vi "Swerve Drive.vi"() -> ()   [LabVIEW 2020]
panel:
  in  "W4 Encoder":dbl
  in  "W3 Encoder":dbl
  in  "W2 Encoder":dbl
  in  "W1 Encoder":dbl
  out "WS 3":dbl
  out "WS 4":dbl
  out "WS 2":dbl
  out "WS 1":dbl
  out "WA 3":dbl
  out "WA 4":dbl
  out "WA 2":dbl
  out "WA 1":dbl
  in  "RCW":dbl(slide) scale=-1.0..1.0
  in  "STR":dbl(slide) scale=-1.0..1.0
  in  "FWD":dbl(slide) scale=-1.0..1.0
  in  "Gyro":dbl
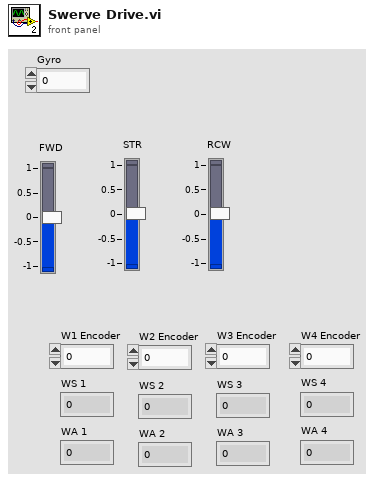
[diagram p1: front panel]
types:
  T1 = typedef "WPI_JoystickDevRef.ctl" = cluster{"Device":T2}
  T2 = typedef "WPI_JoystickDeviceEnum.ctl" = enum16{"USB 0", "USB 1", "USB 2", "USB 3", "USB 4", "USB 5"}
  T3 = typedef "WPI_MotorControlDeviceRef.ctl" = cluster{"DeviceStatus":errorcluster, "Type":T4, "PWM":cluster{"PWM Channel":T5, "DeadBand":T6}, "CAN":cluster{"Device Number":u8, "SetOutput VI Ref":variant, "GetOutput VI Ref":variant, "Enable VI Ref":variant, "Disable VI Ref":variant, "Data":variant}, "Invert":bool, "DIO PWM":cluster{"PWM \"Enable\" Channel":T5, "DIOChannel":T7, "PWM Rate":dbl}}
  T4 = typedef "WPI_MotorControlType.ctl" = enum16{"PWM", "CAN", "DIO PWM"}
  T5 = typedef "FPGA_DIOPWMChannel.ctl" = enum8{"PWM 0", "PWM 1", "PWM 2", "PWM 3", "PWM 4", "PWM 5", "PWM 6", "PWM 7", "PWM 8", "PWM 9", "PWM MXP 0", "PWM MXP 1", "PWM MXP 2", "PWM MXP 3", "PWM MXP 4", "PWM MXP 5", "PWM MXP 6", "PWM MXP 7", "PWM MXP 8", "PWM MXP 9", "Invalid"}
  T6 = typedef "WPI_PWMDeadband.ctl" = cluster{"Name":string, "maxPositivePwm":i32, "minPositivePwm":i32, "centerPwm":i32, "maxNegativePwm":i32, "minNegativePwm":i32, "angularRange":u16}
  T7 = typedef "FPGA_DIOChannel.ctl" = enum8{"DIO 0", "DIO 1", "DIO 2", "DIO 3", "DIO 4", "DIO 5", "DIO 6", "DIO 7", "DIO 8", "DIO 9", "DIO MXP 0", "DIO MXP 1", "DIO MXP 2", "DIO MXP 3", "DIO MXP 4", "DIO MXP 5", "DIO MXP 6", "DIO MXP 7", "DIO MXP 8", "DIO MXP 9", "DIO MXP 10", "DIO MXP 11", "DIO MXP 12", "DIO MXP 13", "DIO MXP 14", "DIO MXP 15", "SPI Port CS1", "SPI Port CS2", "SPI Port CS3", "SPI Port MISO", "SPI Port MOSI", "Invalid"}
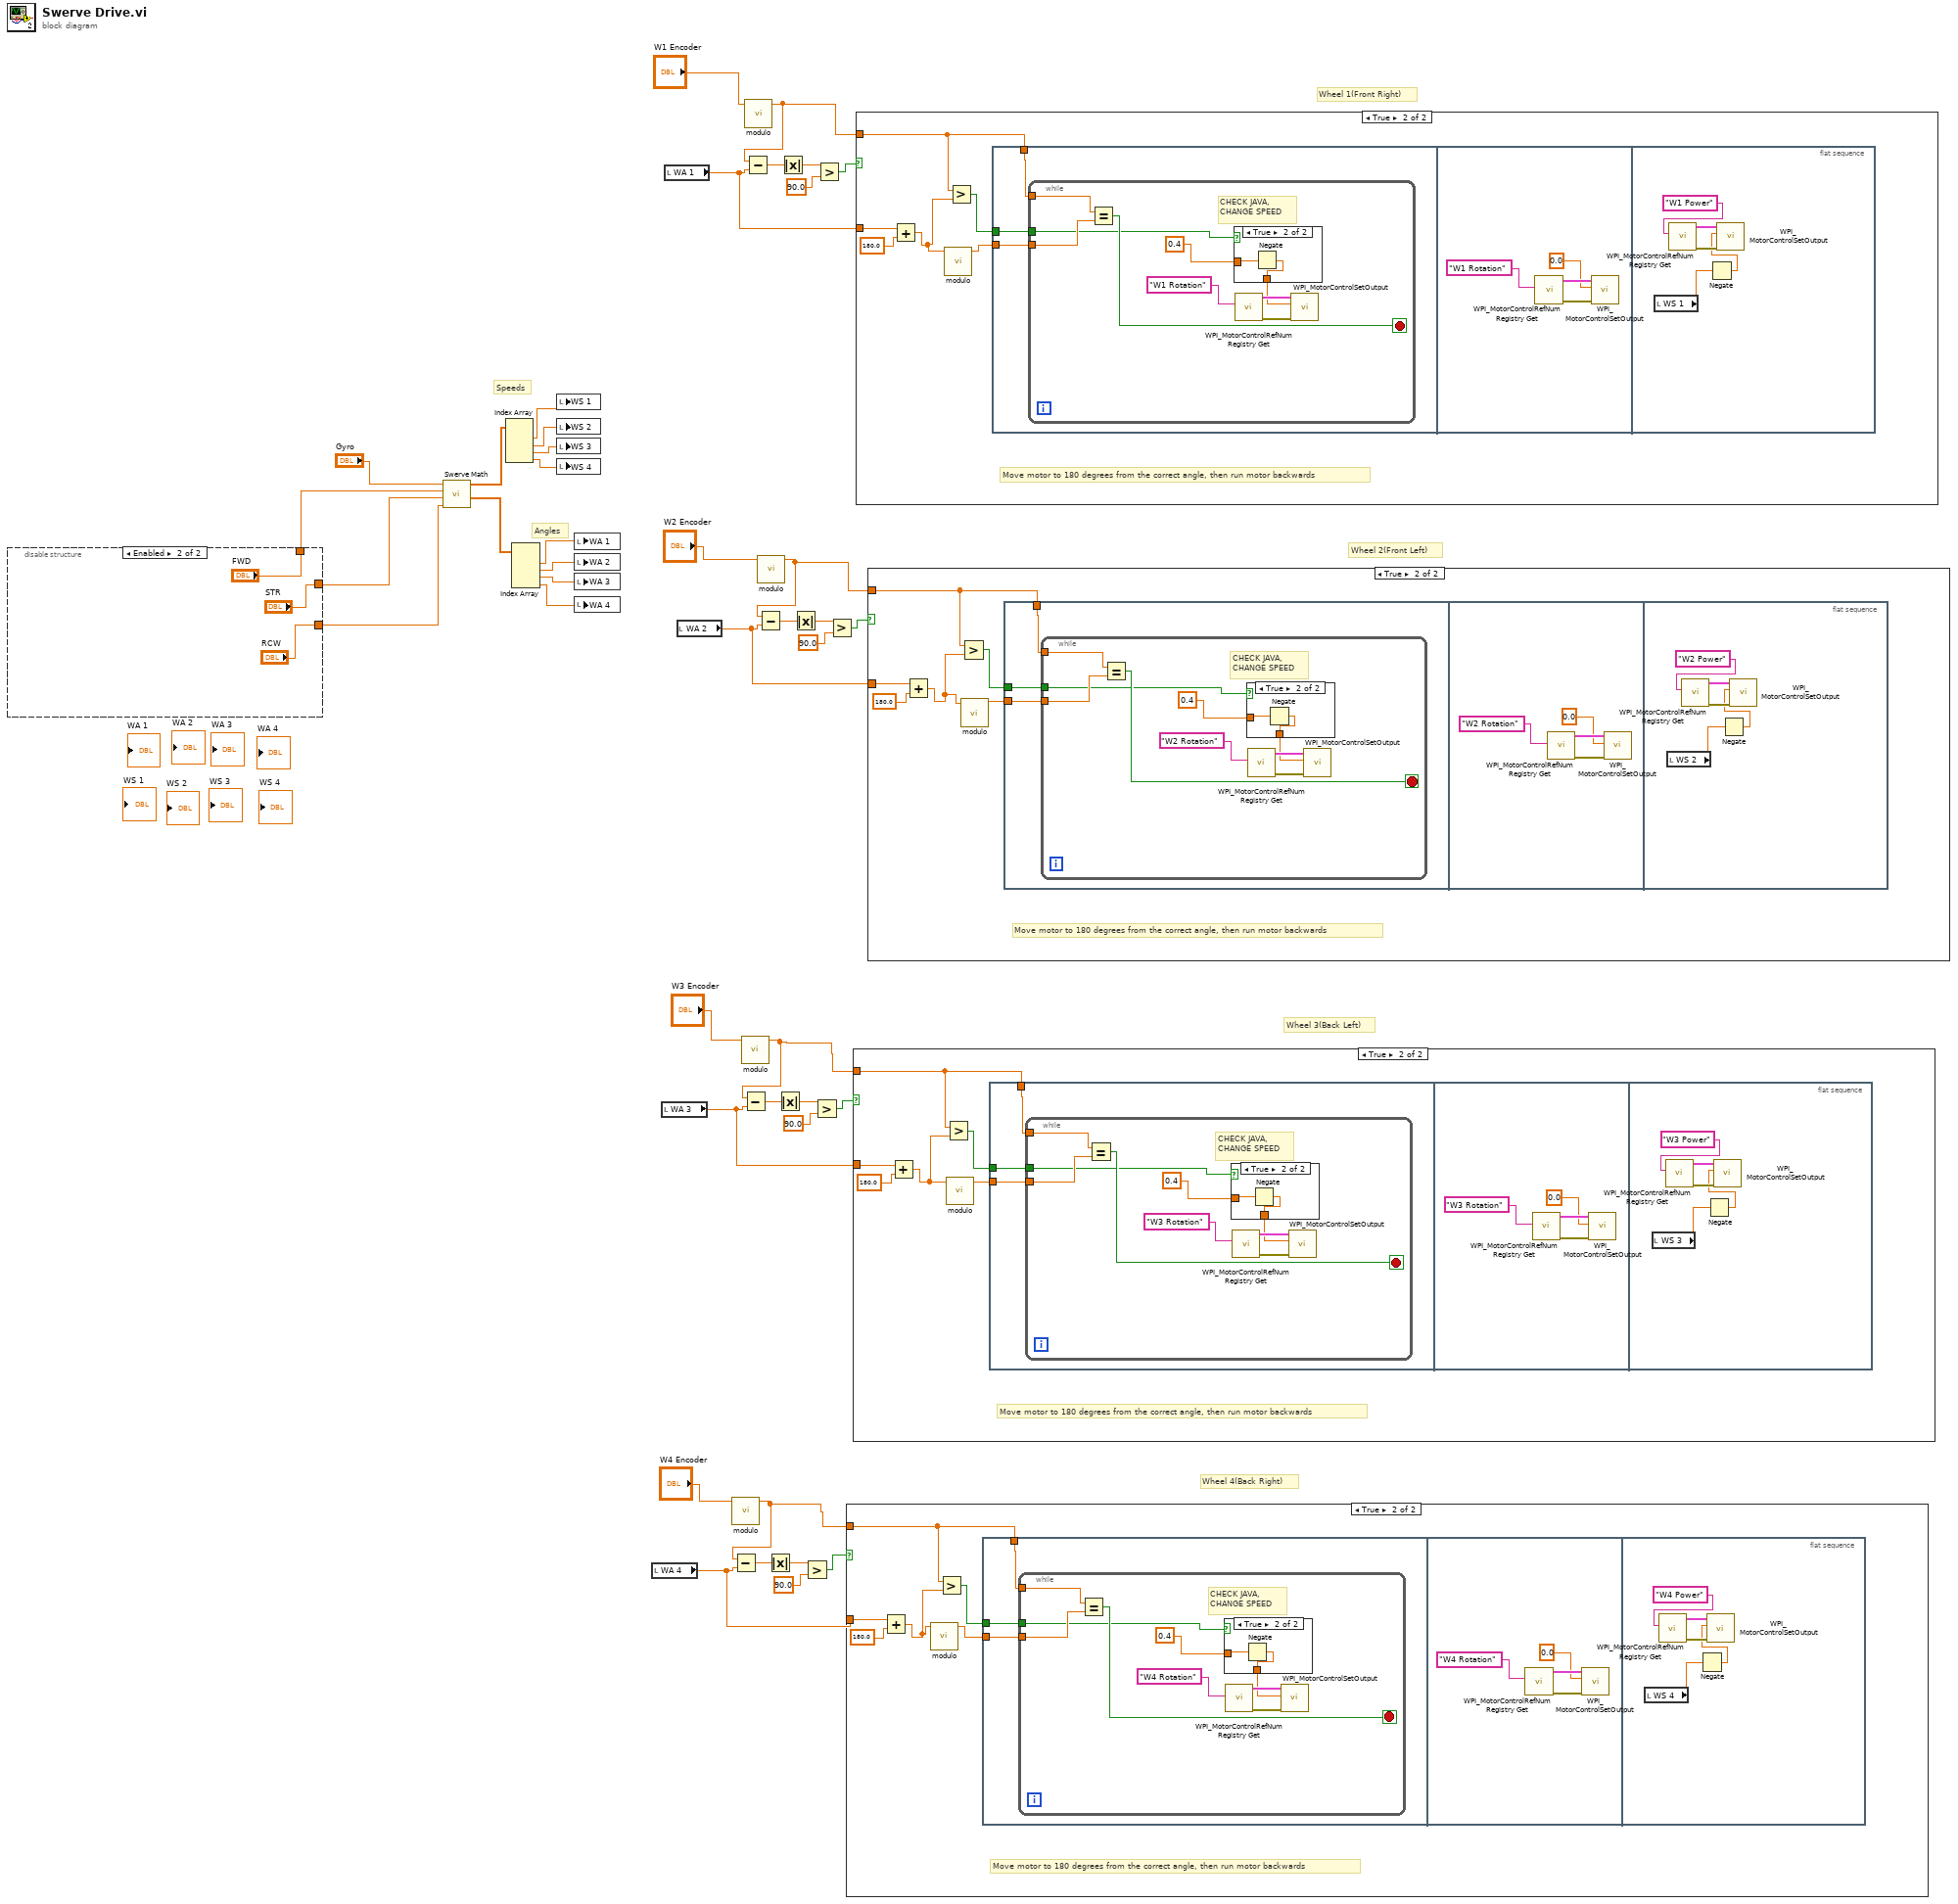
[diagram p0: block diagram]
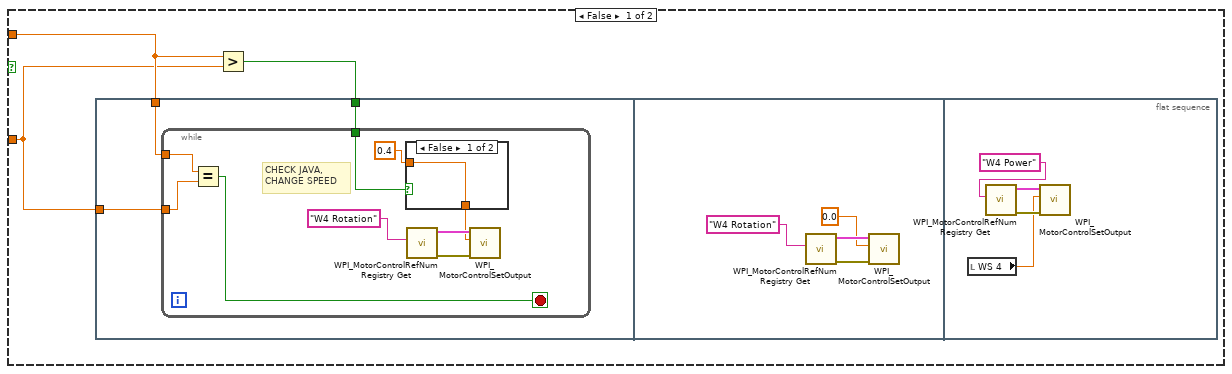
[diagram p2: hidden frame]
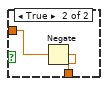
[diagram p3: hidden frame]
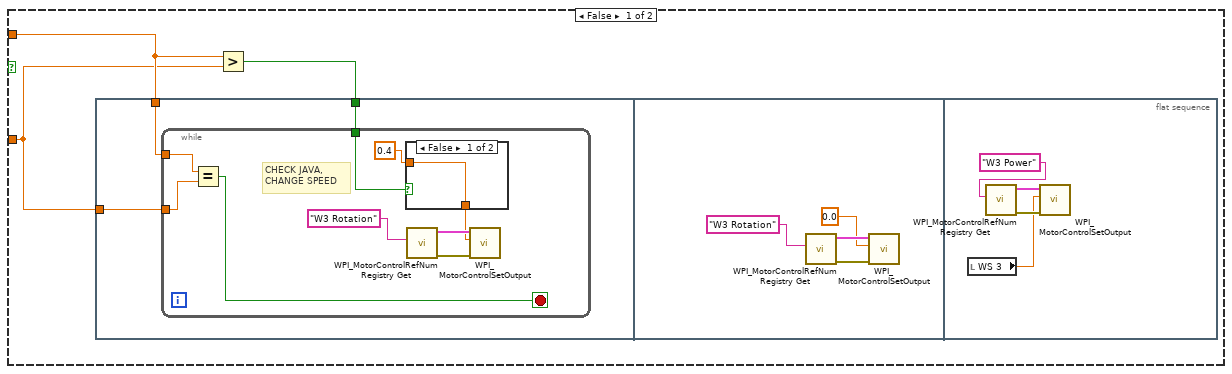
[diagram p5: hidden frame]
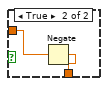
[diagram p6: hidden frame]
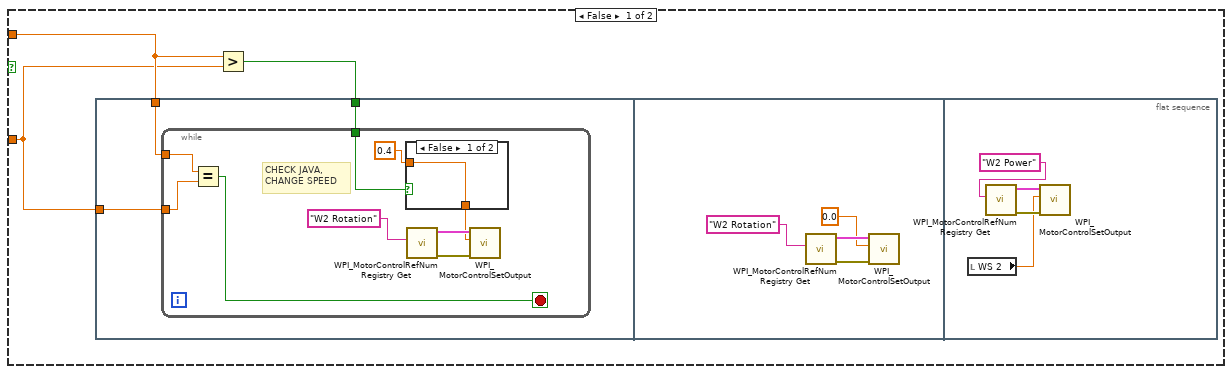
[diagram p8: hidden frame]
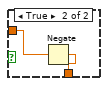
[diagram p9: hidden frame]
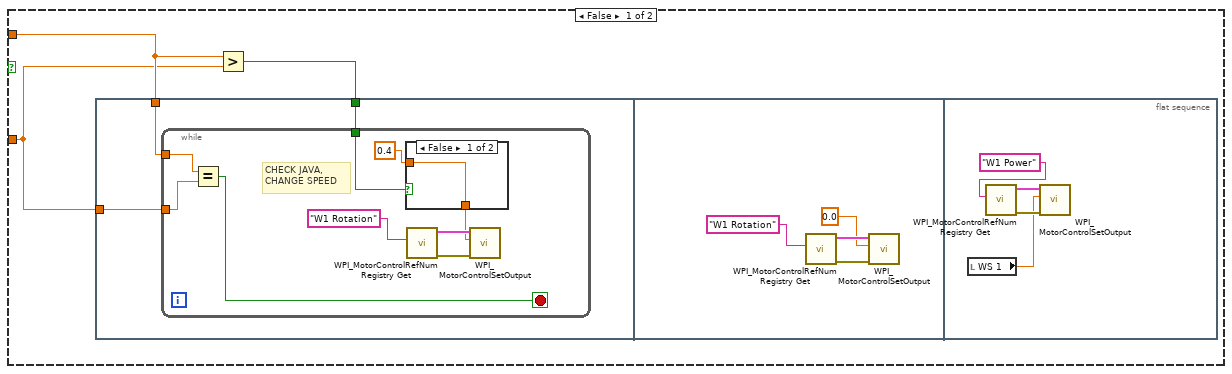
[diagram p11: hidden frame]
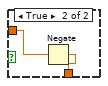
[diagram p12: hidden frame]
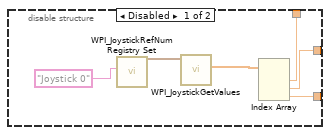
[diagram p14: hidden frame]
diagram:
  # "Wheel 4(Back Right)"
  # "Wheel 3(Back Left)"
  # "Wheel 2(Front Left)"
  # "Wheel 1(Front Right)"
  # "Angles"
  # "Speeds"
  n1 = disable-structure shown="Enabled" {
    disable-tunnel: [w45 "STR"] -> w41
    disable-tunnel: [w44 "RCW"] -> w40
    disable-tunnel: [w43 "FWD"] -> w39
    frame Disabled {
      n2 = call <vilib>:"WPI_JoystickRefNum Registry Set.vi"("refnum name"="Joystick 0") -> ("JoystickDevRef"=w47:T1)  [unwired: 9 in, 1 out]
      n3 = call <vilib>:"WPI_JoystickGetValues.vi"("JoystickDevRef"=w47) -> ("Axes"=w46:dbl[])  [unwired: 6 in, 4 out]
      n4 = Index Array(array=w46) -> (element #1=w43:dbl, element #2=w45:dbl, element #3=w44:dbl)  [unwired: 3 in]
    }
    frame Enabled {
    }
  }
  n5 = call "Swerve Math.vi"("Gyro"="Gyro", "FWD"=w39, "STR"=w41, "RCW"=w40) -> ("Wheel Speeds"=w38:dbl[], "Wheel Angles"=w37:dbl[])  [unwired: 5 in]
  n6 = Index Array(array=w38) -> (element #1=w36:dbl, element #2=w34:dbl, element #3=w35:dbl, element #4=w33:dbl)  [unwired: 4 in]
  n7 = Index Array(array=w37) -> (element #1=w29:dbl, element #2=w30:dbl, element #3=w32:dbl, element #4=w31:dbl)  [unwired: 4 in]
  n8 = local write "WS 1"(w36) -> ()
  n9 = local write "WS 2"(w34) -> ()
  n10 = local write "WS 3"(w35) -> ()
  n11 = local write "WS 4"(w33) -> ()
  n12 = local write "WA 1"(w29) -> ()
  n13 = local write "WA 2"(w30) -> ()
  n14 = local write "WA 3"(w32) -> ()
  n15 = local write "WA 4"(w31) -> ()
  n16 = local read "WA 4"() -> (w3:dbl)
  n17 = local read "WA 3"() -> (w10:dbl)
  n18 = local read "WA 1"() -> (w24:dbl)
  n19 = local read "WA 2"() -> (w17:dbl)
  n20 = call "modulo.vi"("X1"="W4 Encoder") -> ("Result"=w1:dbl)  [unwired: 10 in]
  n21 = Subtract(x=w1, y=w3) -> (x-y=w7:dbl)
  n22 = call "modulo.vi"("X1"="W3 Encoder") -> ("Result"=w8:dbl)  [unwired: 10 in]
  n23 = Subtract(x=w8, y=w10) -> (x-y=w14:dbl)
  n24 = call "modulo.vi"("X1"="W1 Encoder") -> ("Result"=w22:dbl)  [unwired: 10 in]
  n25 = Subtract(x=w22, y=w24) -> (x-y=w28:dbl)
  n26 = call "modulo.vi"("X1"="W2 Encoder") -> ("Result"=w15:dbl)  [unwired: 10 in]
  n27 = Subtract(x=w15, y=w17) -> (x-y=w21:dbl)
  n28 = Absolute Value(x=w7) -> (abs(x)=w6:dbl)
  n29 = Absolute Value(x=w14) -> (abs(x)=w13:dbl)
  n30 = Absolute Value(x=w28) -> (abs(x)=w27:dbl)
  n31 = Absolute Value(x=w21) -> (abs(x)=w20:dbl)
  n32 = Greater?(x=w6, y=90.0) -> (0:w4:bool)
  n33 = Greater?(x=w13, y=90.0) -> (0:w11:bool)
  n34 = Greater?(x=w27, y=90.0) -> (0:w25:bool)
  n35 = Greater?(x=w20, y=90.0) -> (0:w18:bool)
  n36 = case shown="True" w4 {
    tunnel: w3 -> [w53 w83]
    tunnel: w1 -> [w54 w81]
    frame False {
      n37 = flat-sequence {
        tunnel: w54 -> [w57]
        tunnel: w53 -> [w56]
        tunnel: w52 -> [w55]
        frame #0 {
          n38 = while {
            tunnel: w57 -> [w63]
            tunnel: w56 -> [w62]
            tunnel: w55 -> [w58]
            stop <- w61 stop-if-true
            # "CHECK JAVA, \nCHANGE SPEED"
            n39 = Equal?(x=w63, y=w62) -> (x = y?=w61:bool)
            n40 = case shown="False" w58 {
              tunnel: 0.4 ("Output") -> [w67 w69]
              tunnel: [w67 w68] -> w59
              frame False {
              }
              frame True {
                n41 = Negate(x=w69) -> (-x=w68:dbl)
              }
            }
            n42 = call <vilib>:"WPI_MotorControlRefNum Registry Get.vi"("refnum name"="W4 Rotation") -> ("error out"=w65:errorcluster, "MotorControlDevRef"=w66:T3)  [unwired: 9 in]
            n43 = call <vilib>:"WPI_MotorControlSetOutput.vi"("error in (no error)"=w65, "Output"=w59, "MotorControlDevRef"=w66) -> ()  [unwired: 6 in, 3 out]
          }
        }
        frame #1 {
          n44 = call <vilib>:"WPI_MotorControlRefNum Registry Get.vi"("refnum name"="W4 Rotation") -> ("error out"=w72:errorcluster, "MotorControlDevRef"=w73:T3)  [unwired: 9 in]
          n45 = call <vilib>:"WPI_MotorControlSetOutput.vi"("error in (no error)"=w72, "Output"=0.0, "MotorControlDevRef"=w73) -> ()  [unwired: 6 in, 3 out]
        }
        frame #2 {
          n46 = local read "WS 4"() -> (w74:dbl)
          n47 = call <vilib>:"WPI_MotorControlRefNum Registry Get.vi"("refnum name"="W4 Power") -> ("error out"=w76:errorcluster, "MotorControlDevRef"=w75:T3)  [unwired: 9 in]
          n48 = call <vilib>:"WPI_MotorControlSetOutput.vi"("error in (no error)"=w76, "Output"=w74, "MotorControlDevRef"=w75) -> ()  [unwired: 6 in, 3 out]
        }
      }
      n49 = Greater?(x=w54, y=w53) -> (0:w52:bool)
    }
    frame True {
      # "Move motor to 180 degrees from the correct angle, then run motor backwards"
      n50 = Add(x=w83, y=180.0) -> (x+y=w79:dbl)
      n51 = call "modulo.vi"("X1"=w79) -> ("Result"=w78:dbl)  [unwired: 10 in]
      n52 = Greater?(x=w81, y=w79) -> (0:w80:bool)
      n53 = flat-sequence {
        tunnel: w81 -> [w86]
        tunnel: w78 -> [w85]
        tunnel: w80 -> [w84]
        frame #0 {
          n54 = while {
            tunnel: w86 -> [w92]
            tunnel: w85 -> [w91]
            tunnel: w84 -> [w87]
            stop <- w90 stop-if-true
            # "CHECK JAVA, \nCHANGE SPEED"
            n55 = Equal?(x=w92, y=w91) -> (x = y?=w90:bool)
            n56 = case shown="True" w87 {
              tunnel: 0.4 ("Output") -> [w96 w98]
              tunnel: [w96 w97] -> w88
              frame False {
              }
              frame True {
                n57 = Negate(x=w98) -> (-x=w97:dbl)
              }
            }
            n58 = call <vilib>:"WPI_MotorControlRefNum Registry Get.vi"("refnum name"="W4 Rotation") -> ("error out"=w94:errorcluster, "MotorControlDevRef"=w95:T3)  [unwired: 9 in]
            n59 = call <vilib>:"WPI_MotorControlSetOutput.vi"("error in (no error)"=w94, "Output"=w88, "MotorControlDevRef"=w95) -> ()  [unwired: 6 in, 3 out]
          }
        }
        frame #1 {
          n60 = call <vilib>:"WPI_MotorControlRefNum Registry Get.vi"("refnum name"="W4 Rotation") -> ("error out"=w101:errorcluster, "MotorControlDevRef"=w102:T3)  [unwired: 9 in]
          n61 = call <vilib>:"WPI_MotorControlSetOutput.vi"("error in (no error)"=w101, "Output"=0.0, "MotorControlDevRef"=w102) -> ()  [unwired: 6 in, 3 out]
        }
        frame #2 {
          n62 = local read "WS 4"() -> (w103:dbl)
          n63 = call <vilib>:"WPI_MotorControlRefNum Registry Get.vi"("refnum name"="W4 Power") -> ("error out"=w106:errorcluster, "MotorControlDevRef"=w105:T3)  [unwired: 9 in]
          n64 = Negate(x=w103) -> (-x=w104:dbl)
          n65 = call <vilib>:"WPI_MotorControlSetOutput.vi"("error in (no error)"=w106, "Output"=w104, "MotorControlDevRef"=w105) -> ()  [unwired: 6 in, 3 out]
        }
      }
    }
  }
  n66 = case shown="True" w11 {
    tunnel: w10 -> [w109 w139]
    tunnel: w8 -> [w110 w137]
    frame False {
      n67 = flat-sequence {
        tunnel: w110 -> [w113]
        tunnel: w109 -> [w112]
        tunnel: w108 -> [w111]
        frame #0 {
          n68 = while {
            tunnel: w113 -> [w119]
            tunnel: w112 -> [w118]
            tunnel: w111 -> [w114]
            stop <- w117 stop-if-true
            # "CHECK JAVA, \nCHANGE SPEED"
            n69 = Equal?(x=w119, y=w118) -> (x = y?=w117:bool)
            n70 = case shown="False" w114 {
              tunnel: 0.4 ("Output") -> [w123 w125]
              tunnel: [w123 w124] -> w115
              frame False {
              }
              frame True {
                n71 = Negate(x=w125) -> (-x=w124:dbl)
              }
            }
            n72 = call <vilib>:"WPI_MotorControlRefNum Registry Get.vi"("refnum name"="W3 Rotation") -> ("error out"=w121:errorcluster, "MotorControlDevRef"=w122:T3)  [unwired: 9 in]
            n73 = call <vilib>:"WPI_MotorControlSetOutput.vi"("error in (no error)"=w121, "Output"=w115, "MotorControlDevRef"=w122) -> ()  [unwired: 6 in, 3 out]
          }
        }
        frame #1 {
          n74 = call <vilib>:"WPI_MotorControlRefNum Registry Get.vi"("refnum name"="W3 Rotation") -> ("error out"=w128:errorcluster, "MotorControlDevRef"=w129:T3)  [unwired: 9 in]
          n75 = call <vilib>:"WPI_MotorControlSetOutput.vi"("error in (no error)"=w128, "Output"=0.0, "MotorControlDevRef"=w129) -> ()  [unwired: 6 in, 3 out]
        }
        frame #2 {
          n76 = local read "WS 3"() -> (w130:dbl)
          n77 = call <vilib>:"WPI_MotorControlRefNum Registry Get.vi"("refnum name"="W3 Power") -> ("error out"=w132:errorcluster, "MotorControlDevRef"=w131:T3)  [unwired: 9 in]
          n78 = call <vilib>:"WPI_MotorControlSetOutput.vi"("error in (no error)"=w132, "Output"=w130, "MotorControlDevRef"=w131) -> ()  [unwired: 6 in, 3 out]
        }
      }
      n79 = Greater?(x=w110, y=w109) -> (0:w108:bool)
    }
    frame True {
      # "Move motor to 180 degrees from the correct angle, then run motor backwards"
      n80 = Add(x=w139, y=180.0) -> (x+y=w135:dbl)
      n81 = Greater?(x=w137, y=w135) -> (0:w136:bool)
      n82 = call "modulo.vi"("X1"=w135) -> ("Result"=w134:dbl)  [unwired: 10 in]
      n83 = flat-sequence {
        tunnel: w137 -> [w142]
        tunnel: w134 -> [w141]
        tunnel: w136 -> [w140]
        frame #0 {
          n84 = while {
            tunnel: w142 -> [w148]
            tunnel: w141 -> [w147]
            tunnel: w140 -> [w143]
            stop <- w146 stop-if-true
            # "CHECK JAVA, \nCHANGE SPEED"
            n85 = Equal?(x=w148, y=w147) -> (x = y?=w146:bool)
            n86 = case shown="True" w143 {
              tunnel: 0.4 ("Output") -> [w152 w154]
              tunnel: [w152 w153] -> w144
              frame False {
              }
              frame True {
                n87 = Negate(x=w154) -> (-x=w153:dbl)
              }
            }
            n88 = call <vilib>:"WPI_MotorControlRefNum Registry Get.vi"("refnum name"="W3 Rotation") -> ("error out"=w150:errorcluster, "MotorControlDevRef"=w151:T3)  [unwired: 9 in]
            n89 = call <vilib>:"WPI_MotorControlSetOutput.vi"("error in (no error)"=w150, "Output"=w144, "MotorControlDevRef"=w151) -> ()  [unwired: 6 in, 3 out]
          }
        }
        frame #1 {
          n90 = call <vilib>:"WPI_MotorControlRefNum Registry Get.vi"("refnum name"="W3 Rotation") -> ("error out"=w157:errorcluster, "MotorControlDevRef"=w158:T3)  [unwired: 9 in]
          n91 = call <vilib>:"WPI_MotorControlSetOutput.vi"("error in (no error)"=w157, "Output"=0.0, "MotorControlDevRef"=w158) -> ()  [unwired: 6 in, 3 out]
        }
        frame #2 {
          n92 = local read "WS 3"() -> (w159:dbl)
          n93 = call <vilib>:"WPI_MotorControlRefNum Registry Get.vi"("refnum name"="W3 Power") -> ("error out"=w162:errorcluster, "MotorControlDevRef"=w161:T3)  [unwired: 9 in]
          n94 = Negate(x=w159) -> (-x=w160:dbl)
          n95 = call <vilib>:"WPI_MotorControlSetOutput.vi"("error in (no error)"=w162, "Output"=w160, "MotorControlDevRef"=w161) -> ()  [unwired: 6 in, 3 out]
        }
      }
    }
  }
  n96 = case shown="True" w25 {
    tunnel: w24 -> [w165 w195]
    tunnel: w22 -> [w166 w193]
    frame False {
      n97 = flat-sequence {
        tunnel: w166 -> [w169]
        tunnel: w165 -> [w168]
        tunnel: w164 -> [w167]
        frame #0 {
          n98 = while {
            tunnel: w169 -> [w175]
            tunnel: w168 -> [w174]
            tunnel: w167 -> [w170]
            stop <- w173 stop-if-true
            # "CHECK JAVA, \nCHANGE SPEED"
            n99 = Equal?(x=w175, y=w174) -> (x = y?=w173:bool)
            n100 = case shown="False" w170 {
              tunnel: 0.4 ("Output") -> [w179 w181]
              tunnel: [w179 w180] -> w171
              frame False {
              }
              frame True {
                n101 = Negate(x=w181) -> (-x=w180:dbl)
              }
            }
            n102 = call <vilib>:"WPI_MotorControlRefNum Registry Get.vi"("refnum name"="W1 Rotation") -> ("error out"=w177:errorcluster, "MotorControlDevRef"=w178:T3)  [unwired: 9 in]
            n103 = call <vilib>:"WPI_MotorControlSetOutput.vi"("error in (no error)"=w177, "Output"=w171, "MotorControlDevRef"=w178) -> ()  [unwired: 6 in, 3 out]
          }
        }
        frame #1 {
          n104 = call <vilib>:"WPI_MotorControlRefNum Registry Get.vi"("refnum name"="W1 Rotation") -> ("error out"=w184:errorcluster, "MotorControlDevRef"=w185:T3)  [unwired: 9 in]
          n105 = call <vilib>:"WPI_MotorControlSetOutput.vi"("error in (no error)"=w184, "Output"=0.0, "MotorControlDevRef"=w185) -> ()  [unwired: 6 in, 3 out]
        }
        frame #2 {
          n106 = local read "WS 1"() -> (w186:dbl)
          n107 = call <vilib>:"WPI_MotorControlRefNum Registry Get.vi"("refnum name"="W1 Power") -> ("error out"=w188:errorcluster, "MotorControlDevRef"=w187:T3)  [unwired: 9 in]
          n108 = call <vilib>:"WPI_MotorControlSetOutput.vi"("error in (no error)"=w188, "Output"=w186, "MotorControlDevRef"=w187) -> ()  [unwired: 6 in, 3 out]
        }
      }
      n109 = Greater?(x=w166, y=w165) -> (0:w164:bool)
    }
    frame True {
      # "Move motor to 180 degrees from the correct angle, then run motor backwards"
      n110 = Add(x=w195, y=180.0) -> (x+y=w191:dbl)
      n111 = call "modulo.vi"("X1"=w191) -> ("Result"=w190:dbl)  [unwired: 10 in]
      n112 = Greater?(x=w193, y=w191) -> (0:w192:bool)
      n113 = flat-sequence {
        tunnel: w193 -> [w198]
        tunnel: w190 -> [w197]
        tunnel: w192 -> [w196]
        frame #0 {
          n114 = while {
            tunnel: w198 -> [w204]
            tunnel: w197 -> [w203]
            tunnel: w196 -> [w199]
            stop <- w202 stop-if-true
            # "CHECK JAVA, \nCHANGE SPEED"
            n115 = Equal?(x=w204, y=w203) -> (x = y?=w202:bool)
            n116 = case shown="True" w199 {
              tunnel: 0.4 ("Output") -> [w208 w210]
              tunnel: [w208 w209] -> w200
              frame False {
              }
              frame True {
                n117 = Negate(x=w210) -> (-x=w209:dbl)
              }
            }
            n118 = call <vilib>:"WPI_MotorControlRefNum Registry Get.vi"("refnum name"="W1 Rotation") -> ("error out"=w206:errorcluster, "MotorControlDevRef"=w207:T3)  [unwired: 9 in]
            n119 = call <vilib>:"WPI_MotorControlSetOutput.vi"("error in (no error)"=w206, "Output"=w200, "MotorControlDevRef"=w207) -> ()  [unwired: 6 in, 3 out]
          }
        }
        frame #1 {
          n120 = call <vilib>:"WPI_MotorControlRefNum Registry Get.vi"("refnum name"="W1 Rotation") -> ("error out"=w213:errorcluster, "MotorControlDevRef"=w214:T3)  [unwired: 9 in]
          n121 = call <vilib>:"WPI_MotorControlSetOutput.vi"("error in (no error)"=w213, "Output"=0.0, "MotorControlDevRef"=w214) -> ()  [unwired: 6 in, 3 out]
        }
        frame #2 {
          n122 = local read "WS 1"() -> (w215:dbl)
          n123 = call <vilib>:"WPI_MotorControlRefNum Registry Get.vi"("refnum name"="W1 Power") -> ("error out"=w218:errorcluster, "MotorControlDevRef"=w217:T3)  [unwired: 9 in]
          n124 = Negate(x=w215) -> (-x=w216:dbl)
          n125 = call <vilib>:"WPI_MotorControlSetOutput.vi"("error in (no error)"=w218, "Output"=w216, "MotorControlDevRef"=w217) -> ()  [unwired: 6 in, 3 out]
        }
      }
    }
  }
  n126 = case shown="True" w18 {
    tunnel: w17 -> [w221 w251]
    tunnel: w15 -> [w222 w249]
    frame False {
      n127 = flat-sequence {
        tunnel: w222 -> [w225]
        tunnel: w221 -> [w224]
        tunnel: w220 -> [w223]
        frame #0 {
          n128 = while {
            tunnel: w225 -> [w231]
            tunnel: w224 -> [w230]
            tunnel: w223 -> [w226]
            stop <- w229 stop-if-true
            # "CHECK JAVA, \nCHANGE SPEED"
            n129 = Equal?(x=w231, y=w230) -> (x = y?=w229:bool)
            n130 = case shown="False" w226 {
              tunnel: 0.4 ("Output") -> [w235 w237]
              tunnel: [w235 w236] -> w227
              frame False {
              }
              frame True {
                n131 = Negate(x=w237) -> (-x=w236:dbl)
              }
            }
            n132 = call <vilib>:"WPI_MotorControlRefNum Registry Get.vi"("refnum name"="W2 Rotation") -> ("error out"=w233:errorcluster, "MotorControlDevRef"=w234:T3)  [unwired: 9 in]
            n133 = call <vilib>:"WPI_MotorControlSetOutput.vi"("error in (no error)"=w233, "Output"=w227, "MotorControlDevRef"=w234) -> ()  [unwired: 6 in, 3 out]
          }
        }
        frame #1 {
          n134 = call <vilib>:"WPI_MotorControlRefNum Registry Get.vi"("refnum name"="W2 Rotation") -> ("error out"=w240:errorcluster, "MotorControlDevRef"=w241:T3)  [unwired: 9 in]
          n135 = call <vilib>:"WPI_MotorControlSetOutput.vi"("error in (no error)"=w240, "Output"=0.0, "MotorControlDevRef"=w241) -> ()  [unwired: 6 in, 3 out]
        }
        frame #2 {
          n136 = local read "WS 2"() -> (w242:dbl)
          n137 = call <vilib>:"WPI_MotorControlRefNum Registry Get.vi"("refnum name"="W2 Power") -> ("error out"=w244:errorcluster, "MotorControlDevRef"=w243:T3)  [unwired: 9 in]
          n138 = call <vilib>:"WPI_MotorControlSetOutput.vi"("error in (no error)"=w244, "Output"=w242, "MotorControlDevRef"=w243) -> ()  [unwired: 6 in, 3 out]
        }
      }
      n139 = Greater?(x=w222, y=w221) -> (0:w220:bool)
    }
    frame True {
      # "Move motor to 180 degrees from the correct angle, then run motor backwards"
      n140 = Add(x=w251, y=180.0) -> (x+y=w247:dbl)
      n141 = Greater?(x=w249, y=w247) -> (0:w248:bool)
      n142 = call "modulo.vi"("X1"=w247) -> ("Result"=w246:dbl)  [unwired: 10 in]
      n143 = flat-sequence {
        tunnel: w249 -> [w254]
        tunnel: w246 -> [w253]
        tunnel: w248 -> [w252]
        frame #0 {
          n144 = while {
            tunnel: w254 -> [w260]
            tunnel: w253 -> [w259]
            tunnel: w252 -> [w255]
            stop <- w258 stop-if-true
            # "CHECK JAVA, \nCHANGE SPEED"
            n145 = Equal?(x=w260, y=w259) -> (x = y?=w258:bool)
            n146 = case shown="True" w255 {
              tunnel: 0.4 ("Output") -> [w264 w266]
              tunnel: [w264 w265] -> w256
              frame False {
              }
              frame True {
                n147 = Negate(x=w266) -> (-x=w265:dbl)
              }
            }
            n148 = call <vilib>:"WPI_MotorControlRefNum Registry Get.vi"("refnum name"="W2 Rotation") -> ("error out"=w262:errorcluster, "MotorControlDevRef"=w263:T3)  [unwired: 9 in]
            n149 = call <vilib>:"WPI_MotorControlSetOutput.vi"("error in (no error)"=w262, "Output"=w256, "MotorControlDevRef"=w263) -> ()  [unwired: 6 in, 3 out]
          }
        }
        frame #1 {
          n150 = call <vilib>:"WPI_MotorControlRefNum Registry Get.vi"("refnum name"="W2 Rotation") -> ("error out"=w269:errorcluster, "MotorControlDevRef"=w270:T3)  [unwired: 9 in]
          n151 = call <vilib>:"WPI_MotorControlSetOutput.vi"("error in (no error)"=w269, "Output"=0.0, "MotorControlDevRef"=w270) -> ()  [unwired: 6 in, 3 out]
        }
        frame #2 {
          n152 = local read "WS 2"() -> (w271:dbl)
          n153 = call <vilib>:"WPI_MotorControlRefNum Registry Get.vi"("refnum name"="W2 Power") -> ("error out"=w274:errorcluster, "MotorControlDevRef"=w273:T3)  [unwired: 9 in]
          n154 = Negate(x=w271) -> (-x=w272:dbl)
          n155 = call <vilib>:"WPI_MotorControlSetOutput.vi"("error in (no error)"=w274, "Output"=w272, "MotorControlDevRef"=w273) -> ()  [unwired: 6 in, 3 out]
        }
      }
    }
  }
